vi "motor fpga PID test 001.vi"() -> ()   [LabVIEW 2019]
uses:
  motor single class/Motor single.lvclass
  motor enum(FPGA).ctl
  <vilib>/Platform/TimedLoop/XDataNode/timing_clust.ctl
  <vilib>/Platform/TimedLoop/XDataNode/nitl_modes.ctl
  <vilib>/Platform/TimedLoop/XDataNode/wakeup.ctl
  motor single class/Variable PID(Kp).ctl
  motor single class/Variable PID(Kp) mode enum.ctl
  <vilib>/platform/TimedLoop/XDataNode/XDataNode.xnode
  <vilib>/Platform/TimedLoop/XDataNode/XDNodeRunTimeDep.lvlib
panel:
  out "error out 2":errorcluster
  in  "Vertical Pointer Slide 2":dbl(slide) scale=-125.0..125.0
  out "error out":errorcluster
  in  "stop":bool
  in  "Vertical Pointer Slide":dbl(slide) scale=-125.0..125.0
  in  "error in":errorcluster
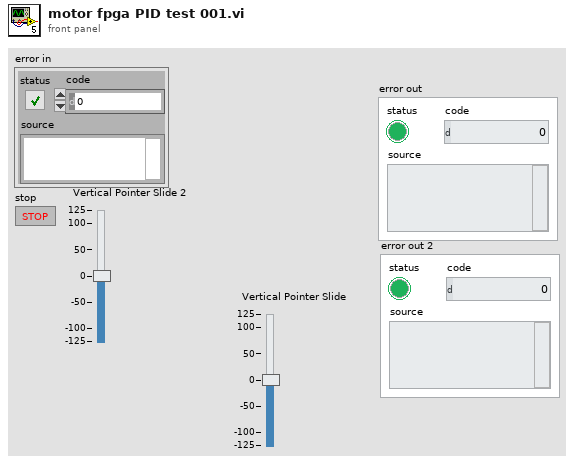
[diagram p1: front panel]
types:
  T1 = typedef "Motor single.lvclass/motor enum(FPGA).ctl" = enum16{"M1", "M2", "M3", "M4"}
  T2 = typedef "Motor single.lvclass/Variable PID(Kp).ctl" = cluster{"Enable variable PID(Kp)":bool, "Variable PID(Kp)range":dbl, "Variable MODE":T3}
  T3 = typedef "Motor single.lvclass/Variable PID(Kp) mode enum.ctl" = enum16{"Log", "Sin&Cos", "Linear", "reverse Log", "const"}
  T4 = typedef "XDNodeRunTimeDep.lvlib/timing_clust.ctl" = cluster{"Expected End [f-1]":u64, "Actual End [f-1]":u64, "Finished Late? [f-1]":bool, "Expected End [i-1]":u64, "Actual End [i-1]":u64, "Finished Late? [i-1]":bool, "Expected Start [i]":u64, "Actual Start [i]":u64, "Expected Start [f]":u64, "Actual Start [f]":u64, "Source Name":string, "Structure Name":string, "Period":i64, "Deadline":i64, "Offset":i64, "Start":i64, "Priority":i32, "Timeout":i32, "Mode":T5, "Wakeup Reason":T6, "Error":errorcluster, "Source Type":string, "Secondary Source Type":string, "Global End Time":u64, "Global Start Time":u64, "Frame Duration":u64, "Iteration Duration":u64, "Assigned CPU":i32, "I/O Scan Engine Mode":u32}
  T5 = typedef "XDNodeRunTimeDep.lvlib/nitl_modes.ctl" = enum32{"No Change", "Process missed periods, maintain original phase", "Discard missed periods, maintain original phase", "Process missed periods, ignore original phase", "Discard missed periods, ignore original phase"}
  T6 = typedef "XDNodeRunTimeDep.lvlib/wakeup.ctl" = enum32{"Normal", "Aborted", "Asynchronous wakeup", "Timing source error", "Timed loop error", "Timeout"}
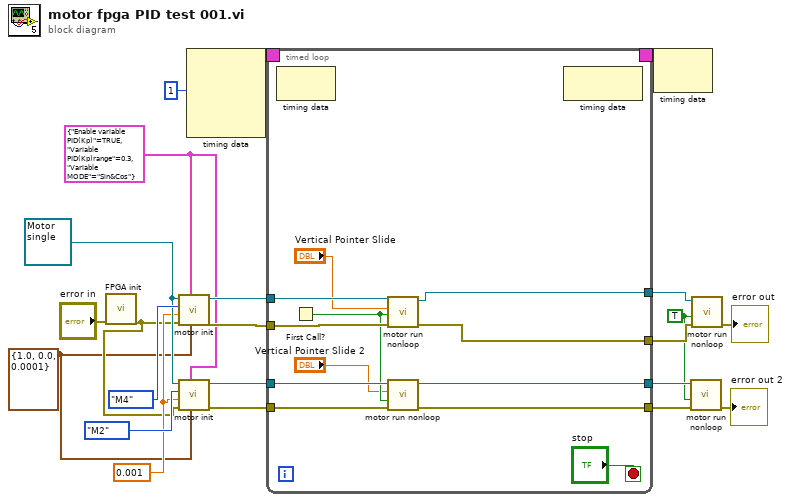
[diagram p0: block diagram]
diagram:
  w2 = TRUE ("Reset")
  w11 = T2 {"Enable variable PID(Kp)"=TRUE, "Variable PID(Kp)range"=0.3, "Variable MODE"=enum."Sin&Cos"} ("Variable PID(Kp)")
  w7 = cluster{"Kp":dbl, "Ki":dbl, "Kd":dbl} {"Kp"=1.0, "Ki"=0.0, "Kd"=0.0001} ("PID")
  w9 = 0.001 ("dt(s)")
  w12 = refnum<class "Motor single.lvclass"> refnum ("Motor single.lvclass")
  n1 = call "FPGA init.vi"("error in"="error in") -> ("error out"=w8:errorcluster)  [unwired: 9 in, 1 out]
  n2 = call "motor init.vi"("PID"=w7, "Variable PID(Kp)"=w11, "Error In"=w8, "dt(s)"=w9, "Enum"=motor_enum(FPGA)."M4", "Motor single.lvclass"=w12) -> ("Error Out"=w17:errorcluster, "output object"=w18:refnum<class "Motor single.lvclass">)  [unwired: 4 in]
  n3 = call "motor init.vi"("PID"=w7, "Variable PID(Kp)"=w11, "Error In"=w8, "dt(s)"=w9, "Enum"=motor_enum(FPGA)."M2", "Motor single.lvclass"=w12) -> ("Error Out"=w6:errorcluster, "output object"=w5:refnum<class "Motor single.lvclass">)  [unwired: 4 in]
  n4 = node-c288(i64 1 ("Period")) -> (w20:T4)  [unwired: 3 in]
  n5 = timed-loop {
    timing: w20 -> [_]
    timing-out: [_] -> w19
    tunnel: w18 -> [w34]
    tunnel: w17 -> [w32]
    tunnel: [w30] -> w15
    tunnel: [w29] -> w14
    tunnel: w6 -> [w28]
    tunnel: w5 -> [w27]
    tunnel: [w24] -> w4
    tunnel: [w23] -> w3
    stop <- "stop" stop-if-true
    n6 = node-c288() -> ()  [unwired: 1 in, 1 out]
    n7 = First Call?() -> (First Call?: T/F=w26:bool)
    n8 = call "motor run nonloop.vi"("Error In"=w32, "Reset"=w26, "Speed (RPM)"="Vertical Pointer Slide", "Motor single.lvclass"=w34) -> ("error out"=w29:errorcluster, "output cluster"=w30:refnum<class "Motor single.lvclass">)  [unwired: 3 in, 3 out]
    n9 = call "motor run nonloop.vi"("Error In"=w28, "Reset"=w26, "Speed (RPM)"="Vertical Pointer Slide 2", "Motor single.lvclass"=w27) -> ("error out"=w24:errorcluster, "output cluster"=w23:refnum<class "Motor single.lvclass">)  [unwired: 3 in, 3 out]
    n10 = node-c288() -> ()  [unwired: 1 in, 1 out]
  }
  n11 = node-c288(w19) -> ()  [unwired: 1 out]
  n12 = call "motor run nonloop.vi"("Error In"=w4, "Reset"=w2, "Motor single.lvclass"=w3) -> ("error out"=→"error out 2":errorcluster)  [unwired: 4 in, 4 out]
  n13 = call "motor run nonloop.vi"("Error In"=w14, "Reset"=w2, "Motor single.lvclass"=w15) -> ("error out"=→"error out":errorcluster)  [unwired: 4 in, 4 out]
